vi "Flat Secuence.vi"() -> ()   [LabVIEW 2020]
panel:
  out "Thermometer 3":u8(slide) scale=0.0..100.0
  out "Thermometer 2":u8(slide) scale=0.0..100.0
  out "Thermometer":u8(slide) scale=0.0..100.0
  # "Flat secuence"
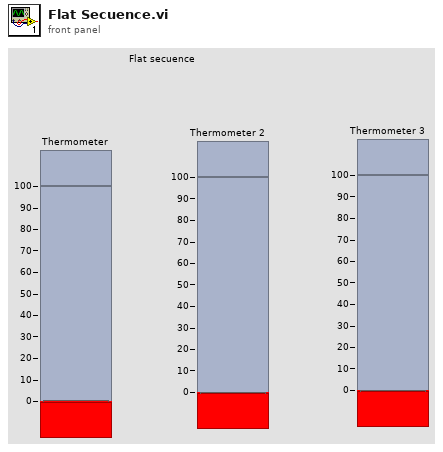
[diagram p1: front panel]
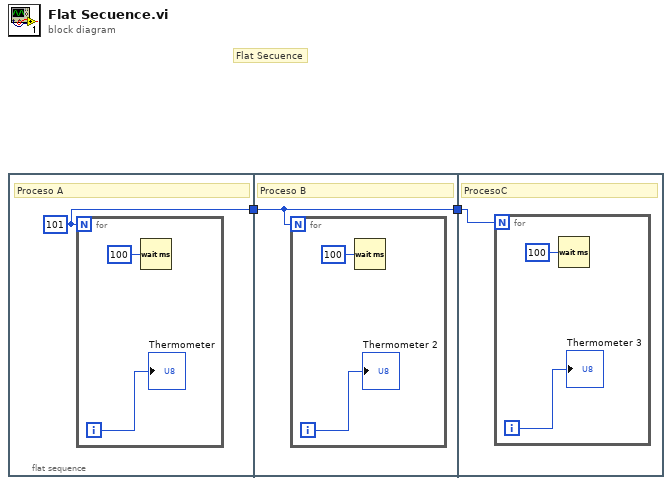
[diagram p0: block diagram]
diagram:
  # "Flat Secuence"
  n1 = flat-sequence {
    tunnel: [w3] -> w2
    tunnel: w2 -> [w6]
    tunnel: [w6] -> w1
    tunnel: w1 -> [w9]
    frame #0 {
      w3 = 101
      # "Proceso A"
      n2 = for {
        N: w3 -> [_]
        i -> [w4]
        n3 = Wait (ms)(milliseconds to wait=u32 100) -> ()  [unwired: 1 out]
        "Thermometer" <- w4
      }
    }
    frame #1 {
      # "Proceso B"
      n4 = for {
        N: w6 -> [_]
        i -> [w7]
        n5 = Wait (ms)(milliseconds to wait=u32 100) -> ()  [unwired: 1 out]
        "Thermometer 2" <- w7
      }
    }
    frame #2 {
      # "ProcesoC"
      n6 = for {
        N: w9 -> [_]
        i -> [w10]
        n7 = Wait (ms)(milliseconds to wait=u32 100) -> ()  [unwired: 1 out]
        "Thermometer 3" <- w10
      }
    }
  }
